vi "Teleop.vi"(10 "Match Info":T1={"Autonomous Elapsed Seconds"=0.0, "TeleOp Elapsed Seconds"=0.0, "Disabled Elapsed Seconds"=0.0, "Visited Autonomous"=FALSE, "Visited TeleOp"=FALSE, "Visited Disabled"=FALSE, "Autonomous Settings"={"Autonomous Style"=enum."Independent", "VI Refnum"=refnum}}, 11 "Call Context":T2) -> ()   [LabVIEW 2017]
doc: "This VI is called for each enabled TeleOp packet received from the DS. It is typically used to read from joysticks and other inputs and update I/O or setpoints for timed control loops. It should complete and return within 20 milliseconds or risk missing DS packets."
uses:
  <vilib>/Rock Robotics/WPI/DriverStation/WPI_DriverStationDerivedRobotMode.ctl
  <vilib>/Rock Robotics/WPI/DriverStation/WPI_DriverStationMatch Info.ctl
  <vilib>/Rock Robotics/WPI/Utilities/WPI_GetSetVariantRefNum.vi
  <vilib>/Rock Robotics/Network Tables/NT Write Boolean Array.vi
  <vilib>/Rock Robotics/Network Tables/NT Write Numeric Array.vi
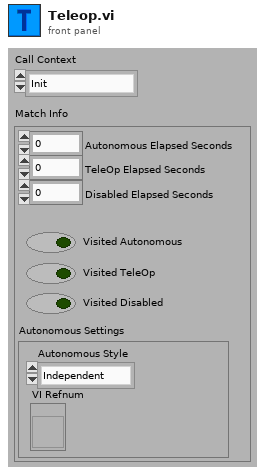
[diagram p1: front panel]
types:
  T1 = typedef "WPI_DriverStationMatch Info.ctl" = cluster{"Autonomous Elapsed Seconds":dbl, "TeleOp Elapsed Seconds":dbl, "Disabled Elapsed Seconds":dbl, "Visited Autonomous":bool, "Visited TeleOp":bool, "Visited Disabled":bool, "Autonomous Settings":cluster{"Autonomous Style":enum16{"Iterative", "Independent"}, "VI Refnum":refnum<vi>}}
  T2 = typedef "WPI_DriverStationDerivedRobotMode.ctl" = enum16{"Init", "Execute", "Stop"}
  T3 = typedef "WPI_JoystickDevRef.ctl" = cluster{"Device":T4}
  T4 = typedef "WPI_JoystickDeviceEnum.ctl" = enum16{"USB 0", "USB 1", "USB 2", "USB 3", "USB 4", "USB 5"}
  T5 = cluster{"Speed Rate":dbl, "Turning Rate":dbl, "Speed Deadband":dbl, "Turning Deadband":dbl, "Square Inputs":bool}
  T6 = typedef "Command Status Info.ctl" = cluster{"Name":string, "Status":T7, "notifier out":T8}
  T7 = typedef "Completion Status.ctl" = enum16{"Successful", "Aborted", "Incomplete"}
  T8 = typedef "Completion Notifier.ctl" = refnum<notifier>
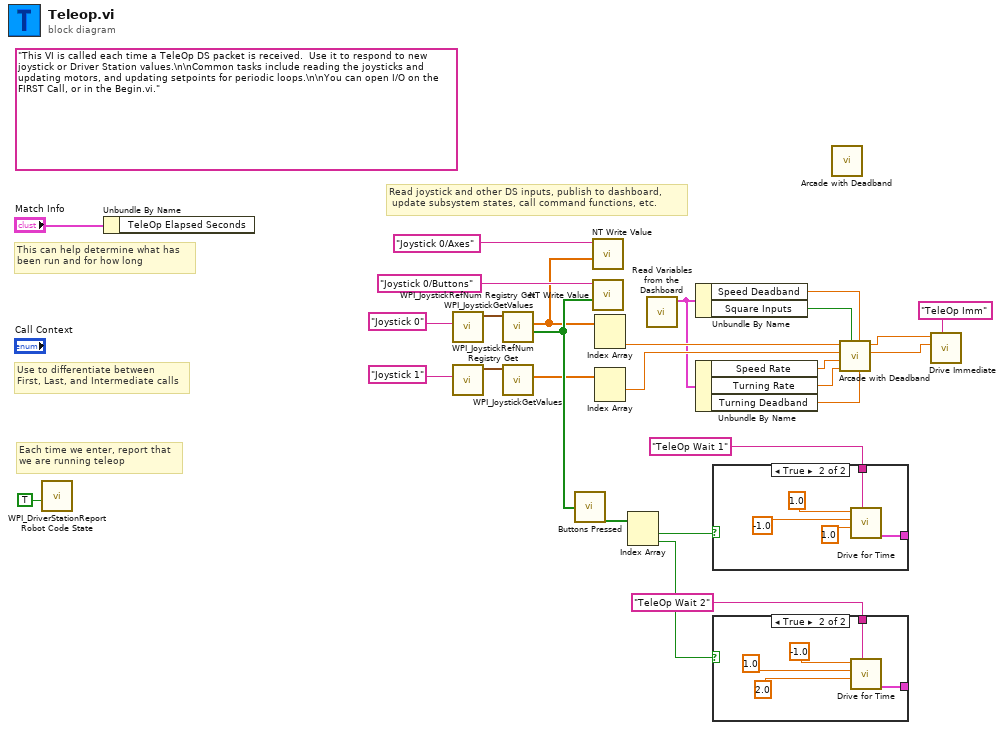
[diagram p0: block diagram]
diagram:
  (unwired) "This VI is called each time a TeleOp DS packet is received.  Use it to respond to new joystick or Driver Station values.\n\nCommon tasks include reading the joysticks and updating motors, and updating setpoints for periodic loops.\n\nYou can open I/O on the FIRST Call, or in the Begin.vi."
  # "Read joystick and other DS inputs, publish to dashboard,\n update subsystem states, call command functions, etc."
  # "Each time we enter, report that\nwe are running teleop"
  # "Use to differentiate between\nFirst, Last, and Intermediate calls"
  # "This can help determine what has\nbeen run and for how long"
  n1 = call <vilib>:"WPI_DriverStationReport Robot Code State.vi"("TeleOp"=TRUE ("Autonomous")) -> ()  [unwired: 10 in, 1 out]
  n2 = Unbundle By Name("Match Info") -> ()  [unwired: 1 out]
  n3 = call <vilib>:"WPI_JoystickRefNum Registry Get.vi"("refnum name"="Joystick 0") -> ("JoystickDevRef"=w24:T3)  [unwired: 1 in, 9 out]
  n4 = call <vilib>:"WPI_JoystickRefNum Registry Get.vi"("refnum name"="Joystick 1") -> ("JoystickDevRef"=w12:T3)  [unwired: 1 in, 9 out]
  n5 = call <vilib>:"WPI_JoystickGetValues.vi"("JoystickDevRef"=w24) -> ("Buttons"=w16:bool[], "Axes"=w15:dbl[])  [unwired: 6 in, 3 out]
  n6 = call <vilib>:"WPI_JoystickGetValues.vi"("JoystickDevRef"=w12) -> ("Axes"=w13:dbl[])  [unwired: 6 in, 4 out]
  n7 = call "Buttons Pressed.vi"("Button Values"=w16) -> ("Button Presses"=w20:bool[])
  n8 = call-poly <vilib>:"NT Write Value.vi"("Numeric Array"=w15, "Name"="Joystick 0/Axes") -> ()  [unwired: 9 in, 1 out]
  n9 = call-poly <vilib>:"NT Write Value.vi"("Boolean Array"=w16, "Name"="Joystick 0/Buttons") -> ()  [unwired: 9 in, 1 out]
  n10 = Index Array(array=w15) -> (element #2=w10:dbl)  [unwired: 2 in, 1 out]
  n11 = Index Array(array=w13) -> (element #1=w9:dbl)  [unwired: 2 in, 1 out]
  n12 = Index Array(array=w20) -> (element #1=w19:bool, element #2=w18:bool)  [unwired: 2 in]
  n13 = call "Read Variables from the Dashboard.vi"() -> ("Dashboard Values"=w4:T5)  [unwired: 11 in]
  n14 = Unbundle By Name(w4) -> ("Speed Deadband"=w6:dbl, "Square Inputs"=w5:bool)
  n15 = Unbundle By Name(w4) -> ("Speed Rate"=w3:dbl, "Turning Rate"=w2:dbl, "Turning Deadband"=w1:dbl)
  n16 = case shown="True" w19 {
    tunnel: [_ w31] -> _
    tunnel: "TeleOp Wait 1" ("Description") -> [_ w30]
    frame False {
    }
    frame True {
      n17 = call "Drive for Time.vi"("Description"=w30, "Seconds"=1.0, "Right Speed"=-1.0, "Left Speed"=1.0) -> ("Command Info Out"=w31:T6)  [unwired: 6 in, 1 out]
    }
  }
  n18 = case shown="True" w18 {
    tunnel: [_ w35] -> _
    tunnel: "TeleOp Wait 2" ("Description") -> [_ w34]
    frame False {
    }
    frame True {
      n19 = call "Drive for Time.vi"("Description"=w34, "Seconds"=2.0, "Right Speed"=1.0, "Left Speed"=-1.0) -> ("Command Info Out"=w35:T6)  [unwired: 6 in, 1 out]
    }
  }
  n20 = call "Arcade with Deadband.vi"() -> ()  [unwired: 10 in, 2 out]
  n21 = call "Arcade with Deadband.vi"("Turning Deadband"=w1, "Speed Deadband"=w6, "Square Inputs"=w5, "Turning Rate"=w2, "Speed Rate"=w3, "Turning Setpoint"=w9, "Speed Setpoint"=w10) -> ("Right Motor Value"=w7:dbl, "Left Motor Value"=w8:dbl)  [unwired: 3 in]
  n22 = call "Drive Immediate.vi"("Description"="TeleOp Imm", "Turning Setpoint"=w7, "Speed Setpoint"=w8) -> ()  [unwired: 8 in, 1 out]
